vi "fetch frame gige DB1605.vi"() -> ()   [LabVIEW 2015]
uses:
  <vilib>/Utility/miscctls.llb/LV3DPointTypeDef.ctl
  <vilib>/Utility/miscctls.llb/LVRGBAColorTypeDef.ctl
  <vilib>/Utility/importsl/GetValueByPointer/datatype.ctl
  <vilib>/Utility/importsl/GetValueByPointer/GetValueByPointer.xnode
  <userlib>/Mv3dRgbd/Mv3dRgbd.lvlib
  <vilib>/picture/3D Picture Control/NI_3D Picture Control.lvlib
  <userlib>/Mv3dRgbdEx/Mv3dRgbdEx.lvlib
panel:
  in  "InputType":cluster{string}
  out "Output":cluster{string}
  out "pstCalibInfo out":T1
  out "handle out":u32
  out "function return":i32
  in  "nCoordinateType":u32
  out "pDeviceCount out 4":u32
  out "pstGigeDeviceInfo out 3":T2
  out "start handle out":u32
  in  "?":enum32{"RGBD", "点云"}(tab)
  out "二维图片":picture
  out "Depth":i16[][](graph)
  out "init function":i32
  out "get list return 3":i32
  out "open gige function 2":i32
  out "start function 2":i32
  out "fetchframe function":i32
  out "stop function":i32
  out "depthtocloud return":i32
  out "close function":i32
  out "release function":i32
  in  "?":bool
  out "MV3D_RGBD_GigEDEVICE_INFO out 3":T3(array[cluster])
  in  "设备索引":i32=5
  out "?":refnum<vi>(3d-picture)
  in  "Name":string="XYZ轴" caption="名称"
  out "大小":i32
  out "x+1":i32
  out "close handle out":u32
  out "stop handle out":u32
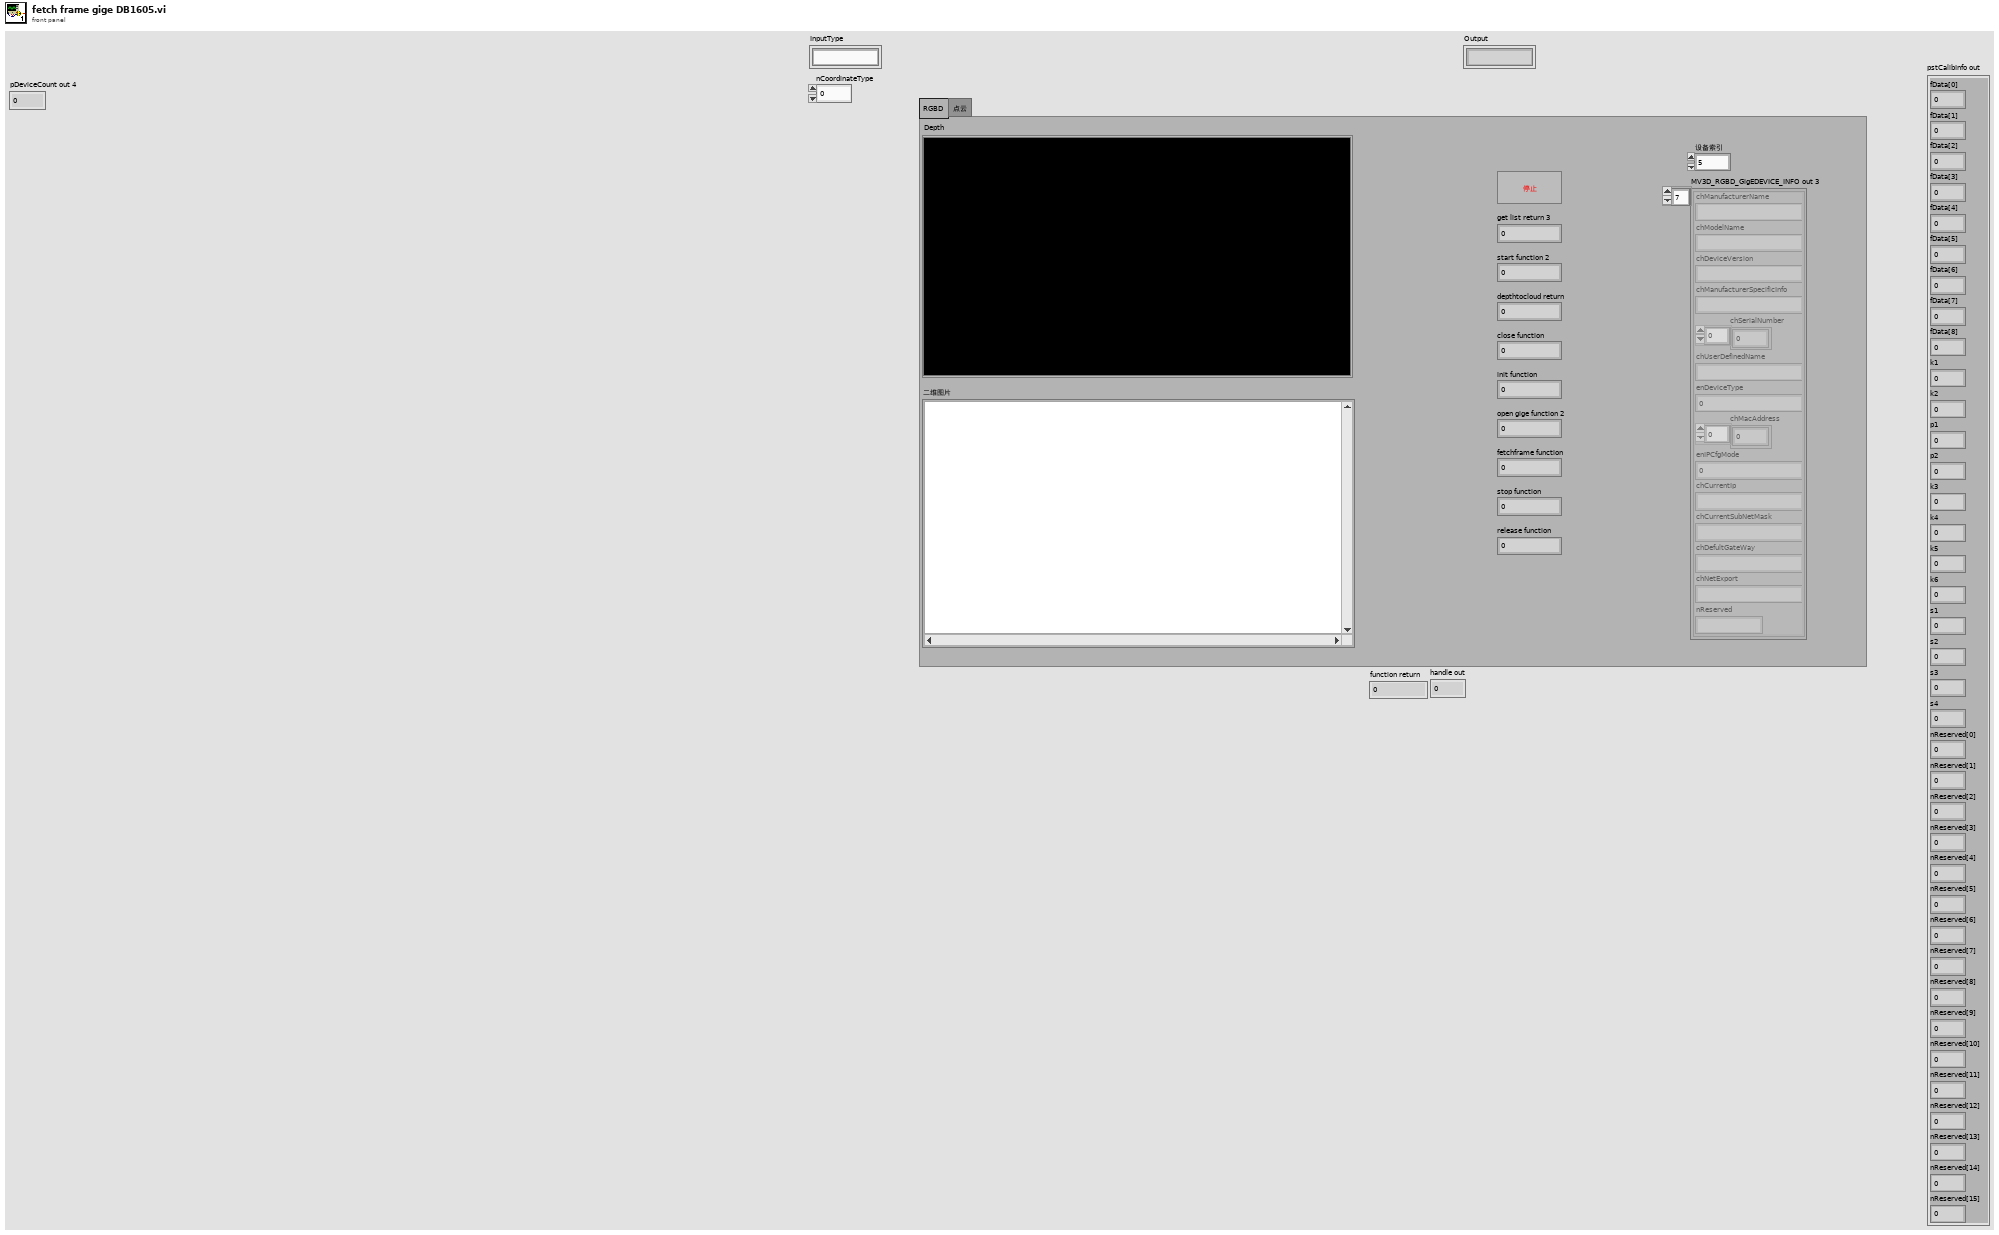
[diagram p1: front panel]
types:
  T1 = cluster{"fData[0]":sgl, "fData[1]":sgl, "fData[2]":sgl, "fData[3]":sgl, "fData[4]":sgl, "fData[5]":sgl, "fData[6]":sgl, "fData[7]":sgl, "fData[8]":sgl, "k1":sgl, "k2":sgl, "p1":sgl, "p2":sgl, "k3":sgl, "k4":sgl, "k5":sgl, "k6":sgl, "s1":sgl, "s2":sgl, "s3":sgl, "s4":sgl, "nReserved[0]":u8, "nReserved[1]":u8, "nReserved[2]":u8, "nReserved[3]":u8, "nReserved[4]":u8, "nReserved[5]":u8, "nReserved[6]":u8, "nReserved[7]":u8, "nReserved[8]":u8, "nReserved[9]":u8, "nReserved[10]":u8, "nReserved[11]":u8, "nReserved[12]":u8, "nReserved[13]":u8, "nReserved[14]":u8, "nReserved[15]":u8}
  T2 = cluster{"chManufacturerName[0]":i8, "chManufacturerName[1]":i8, "chManufacturerName[2]":i8, "chManufacturerName[3]":i8, "chManufacturerName[4]":i8, "chManufacturerName[5]":i8, "chManufacturerName[6]":i8, "chManufacturerName[7]":i8, "chManufacturerName[8]":i8, "chManufacturerName[9]":i8, "chManufacturerName[10]":i8, "chManufacturerName[11]":i8, "chManufacturerName[12]":i8, "chManufacturerName[13]":i8, "chManufacturerName[14]":i8, "chManufacturerName[15]":i8, "chManufacturerName[16]":i8, "chManufacturerName[17]":i8, "chManufacturerName[18]":i8, "chManufacturerName[19]":i8, "chManufacturerName[20]":i8, "chManufacturerName[21]":i8, "chManufacturerName[22]":i8, "chManufacturerName[23]":i8, "chManufacturerName[24]":i8, "chManufacturerName[25]":i8, "chManufacturerName[26]":i8, "chManufacturerName[27]":i8, "chManufacturerName[28]":i8, "chManufacturerName[29]":i8, "chManufacturerName[30]":i8, "chManufacturerName[31]":i8, "chModelName[0]":i8, "chModelName[1]":i8, "chModelName[2]":i8, "chModelName[3]":i8, "chModelName[4]":i8, "chModelName[5]":i8, "chModelName[6]":i8, "chModelName[7]":i8, "chModelName[8]":i8, "chModelName[9]":i8, "chModelName[10]":i8, "chModelName[11]":i8, "chModelName[12]":i8, "chModelName[13]":i8, "chModelName[14]":i8, "chModelName[15]":i8, "chModelName[16]":i8, "chModelName[17]":i8, "chModelName[18]":i8, "chModelName[19]":i8, "chModelName[20]":i8, "chModelName[21]":i8, "chModelName[22]":i8, "chModelName[23]":i8, "chModelName[24]":i8, "chModelName[25]":i8, "chModelName[26]":i8, "chModelName[27]":i8, "chModelName[28]":i8, "chModelName[29]":i8, "chModelName[30]":i8, "chModelName[31]":i8, "chDeviceVersion[0]":i8, "chDeviceVersion[1]":i8, "chDeviceVersion[2]":i8, "chDeviceVersion[3]":i8, "chDeviceVersion[4]":i8, "chDeviceVersion[5]":i8, "chDeviceVersion[6]":i8, "chDeviceVersion[7]":i8, "chDeviceVersion[8]":i8, "chDeviceVersion[9]":i8, "chDeviceVersion[10]":i8, "chDeviceVersion[11]":i8, "chDeviceVersion[12]":i8, "chDeviceVersion[13]":i8, "chDeviceVersion[14]":i8, "chDeviceVersion[15]":i8, "chDeviceVersion[16]":i8, "chDeviceVersion[17]":i8, "chDeviceVersion[18]":i8, "chDeviceVersion[19]":i8, "chDeviceVersion[20]":i8, "chDeviceVersion[21]":i8, "chDeviceVersion[22]":i8, "chDeviceVersion[23]":i8, "chDeviceVersion[24]":i8, "chDeviceVersion[25]":i8, "chDeviceVersion[26]":i8, "chDeviceVersion[27]":i8, "chDeviceVersion[28]":i8, "chDeviceVersion[29]":i8, "chDeviceVersion[30]":i8, "chDeviceVersion[31]":i8, "chManufacturerSpecificInfo[0]":i8, "chManufacturerSpecificInfo[1]":i8, "chManufacturerSpecificInfo[2]":i8, "chManufacturerSpecificInfo[3]":i8, "chManufacturerSpecificInfo[4]":i8, "chManufacturerSpecificInfo[5]":i8, "chManufacturerSpecificInfo[6]":i8, "chManufacturerSpecificInfo[7]":i8, "chManufacturerSpecificInfo[8]":i8, "chManufacturerSpecificInfo[9]":i8, "chManufacturerSpecificInfo[10]":i8, "chManufacturerSpecificInfo[11]":i8, "chManufacturerSpecificInfo[12]":i8, "chManufacturerSpecificInfo[13]":i8, "chManufacturerSpecificInfo[14]":i8, "chManufacturerSpecificInfo[15]":i8, "chManufacturerSpecificInfo[16]":i8, "chManufacturerSpecificInfo[17]":i8, "chManufacturerSpecificInfo[18]":i8, "chManufacturerSpecificInfo[19]":i8, "chManufacturerSpecificInfo[20]":i8, "chManufacturerSpecificInfo[21]":i8, "chManufacturerSpecificInfo[22]":i8, "chManufacturerSpecificInfo[23]":i8, "chManufacturerSpecificInfo[24]":i8, "chManufacturerSpecificInfo[25]":i8, "chManufacturerSpecificInfo[26]":i8, "chManufacturerSpecificInfo[27]":i8, "chManufacturerSpecificInfo[28]":i8, "chManufacturerSpecificInfo[29]":i8, "chManufacturerSpecificInfo[30]":i8, "chManufacturerSpecificInfo[31]":i8, "chManufacturerSpecificInfo[32]":i8, "chManufacturerSpecificInfo[33]":i8, "chManufacturerSpecificInfo[34]":i8, "chManufacturerSpecificInfo[35]":i8, "chManufacturerSpecificInfo[36]":i8, "chManufacturerSpecificInfo[37]":i8, "chManufacturerSpecificInfo[38]":i8, "chManufacturerSpecificInfo[39]":i8, "chManufacturerSpecificInfo[40]":i8, "chManufacturerSpecificInfo[41]":i8, "chManufacturerSpecificInfo[42]":i8, "chManufacturerSpecificInfo[43]":i8, "chManufacturerSpecificInfo[44]":i8, "chManufacturerSpecificInfo[45]":i8, "chManufacturerSpecificInfo[46]":i8, "chManufacturerSpecificInfo[47]":i8, "chSerialNumber[0]":i8, "chSerialNumber[1]":i8, "chSerialNumber[2]":i8, "chSerialNumber[3]":i8, "chSerialNumber[4]":i8, "chSerialNumber[5]":i8, "chSerialNumber[6]":i8, "chSerialNumber[7]":i8, "chSerialNumber[8]":i8, "chSerialNumber[9]":i8, "chSerialNumber[10]":i8, "chSerialNumber[11]":i8, "chSerialNumber[12]":i8, "chSerialNumber[13]":i8, "chSerialNumber[14]":i8, "chSerialNumber[15]":i8, "chUserDefinedName[0]":i8, "chUserDefinedName[1]":i8, "chUserDefinedName[2]":i8, "chUserDefinedName[3]":i8, "chUserDefinedName[4]":i8, "chUserDefinedName[5]":i8, "chUserDefinedName[6]":i8, "chUserDefinedName[7]":i8, "chUserDefinedName[8]":i8, "chUserDefinedName[9]":i8, "chUserDefinedName[10]":i8, "chUserDefinedName[11]":i8, "chUserDefinedName[12]":i8, "chUserDefinedName[13]":i8, "chUserDefinedName[14]":i8, "chUserDefinedName[15]":i8, "enDeviceType":i32, "chMacAddress[0]":u8, "chMacAddress[1]":u8, "chMacAddress[2]":u8, "chMacAddress[3]":u8, "chMacAddress[4]":u8, "chMacAddress[5]":u8, "chMacAddress[6]":u8, "chMacAddress[7]":u8, "enIPCfgMode":i32, "chCurrentIp[0]":i8, "chCurrentIp[1]":i8, "chCurrentIp[2]":i8, "chCurrentIp[3]":i8, "chCurrentIp[4]":i8, "chCurrentIp[5]":i8, "chCurrentIp[6]":i8, "chCurrentIp[7]":i8, "chCurrentIp[8]":i8, "chCurrentIp[9]":i8, "chCurrentIp[10]":i8, "chCurrentIp[11]":i8, "chCurrentIp[12]":i8, "chCurrentIp[13]":i8, "chCurrentIp[14]":i8, "chCurrentIp[15]":i8, "chCurrentSubNetMask[0]":i8, "chCurrentSubNetMask[1]":i8, "chCurrentSubNetMask[2]":i8, "chCurrentSubNetMask[3]":i8, "chCurrentSubNetMask[4]":i8, "chCurrentSubNetMask[5]":i8, "chCurrentSubNetMask[6]":i8, "chCurrentSubNetMask[7]":i8, "chCurrentSubNetMask[8]":i8, "chCurrentSubNetMask[9]":i8, "chCurrentSubNetMask[10]":i8, "chCurrentSubNetMask[11]":i8, "chCurrentSubNetMask[12]":i8, "chCurrentSubNetMask[13]":i8, "chCurrentSubNetMask[14]":i8, "chCurrentSubNetMask[15]":i8, "chDefultGateWay[0]":i8, "chDefultGateWay[1]":i8, "chDefultGateWay[2]":i8, "chDefultGateWay[3]":i8, "chDefultGateWay[4]":i8, "chDefultGateWay[5]":i8, "chDefultGateWay[6]":i8, "chDefultGateWay[7]":i8, "chDefultGateWay[8]":i8, "chDefultGateWay[9]":i8, "chDefultGateWay[10]":i8, "chDefultGateWay[11]":i8, "chDefultGateWay[12]":i8, "chDefultGateWay[13]":i8, "chDefultGateWay[14]":i8, "chDefultGateWay[15]":i8, "chNetExport[0]":i8, "chNetExport[1]":i8, "chNetExport[2]":i8, "chNetExport[3]":i8, "chNetExport[4]":i8, "chNetExport[5]":i8, "chNetExport[6]":i8, "chNetExport[7]":i8, "chNetExport[8]":i8, "chNetExport[9]":i8, "chNetExport[10]":i8, "chNetExport[11]":i8, "chNetExport[12]":i8, "chNetExport[13]":i8, "chNetExport[14]":i8, "chNetExport[15]":i8, "nReserved[0]":u8, "nReserved[1]":u8, "nReserved[2]":u8, "nReserved[3]":u8, "nReserved[4]":u8, "nReserved[5]":u8, "nReserved[6]":u8, "nReserved[7]":u8, "nReserved[8]":u8, "nReserved[9]":u8, "nReserved[10]":u8, "nReserved[11]":u8, "nReserved[12]":u8, "nReserved[13]":u8, "nReserved[14]":u8, "nReserved[15]":u8}
  T3 = cluster{"chManufacturerName":string, "chModelName":string, "chDeviceVersion":string, "chManufacturerSpecificInfo":string, "chSerialNumber":u8[], "chUserDefinedName":string, "enDeviceType":i32, "chMacAddress":u8[], "enIPCfgMode":i32, "chCurrentIp":string, "chCurrentSubNetMask":string, "chDefultGateWay":string, "chNetExport":string, "nReserved":string}[]
  T4 = typedef "LV3DPointTypeDef.ctl" = cluster{"X":sgl, "Y":sgl, "Z":sgl}
  T5 = typedef "LVRGBAColorTypeDef.ctl" = cluster{"Red":sgl, "Green":sgl, "Blue":sgl, "Alpha":sgl}
  T6 = cluster{"Red":sgl, "Green":sgl, "Blue":sgl, "Alpha":sgl}
  T7 = enum32{"pack1", "pack2", "pack4", "pack8", "pack16"}
  T8 = enum16{"Overall", "Per Primitive", "Per Vertex", "Binding Off"}
  T9 = enum16{"Points", "Lines", "Line Strip", "Line Loop", "Triangles", "Triangle Strip", "Triangle Fan", "Quads", "Quad Strip", "Polygon"}
  T10 = cluster{"chManufacturerName[0]":i8, "chManufacturerName[1]":i8, "chManufacturerName[2]":i8, "chManufacturerName[3]":i8, "chManufacturerName[4]":i8, "chManufacturerName[5]":i8, "chManufacturerName[6]":i8, "chManufacturerName[7]":i8, "chManufacturerName[8]":i8, "chManufacturerName[9]":i8, "chManufacturerName[10]":i8, "chManufacturerName[11]":i8, "chManufacturerName[12]":i8, "chManufacturerName[13]":i8, "chManufacturerName[14]":i8, "chManufacturerName[15]":i8, "chManufacturerName[16]":i8, "chManufacturerName[17]":i8, "chManufacturerName[18]":i8, "chManufacturerName[19]":i8, "chManufacturerName[20]":i8, "chManufacturerName[21]":i8, "chManufacturerName[22]":i8, "chManufacturerName[23]":i8, "chManufacturerName[24]":i8, "chManufacturerName[25]":i8, "chManufacturerName[26]":i8, "chManufacturerName[27]":i8, "chManufacturerName[28]":i8, "chManufacturerName[29]":i8, "chManufacturerName[30]":i8, "chManufacturerName[31]":i8, "chModelName[0]":i8, "chModelName[1]":i8, "chModelName[2]":i8, "chModelName[3]":i8, "chModelName[4]":i8, "chModelName[5]":i8, "chModelName[6]":i8, "chModelName[7]":i8, "chModelName[8]":i8, "chModelName[9]":i8, "chModelName[10]":i8, "chModelName[11]":i8, "chModelName[12]":i8, "chModelName[13]":i8, "chModelName[14]":i8, "chModelName[15]":i8, "chModelName[16]":i8, "chModelName[17]":i8, "chModelName[18]":i8, "chModelName[19]":i8, "chModelName[20]":i8, "chModelName[21]":i8, "chModelName[22]":i8, "chModelName[23]":i8, "chModelName[24]":i8, "chModelName[25]":i8, "chModelName[26]":i8, "chModelName[27]":i8, "chModelName[28]":i8, "chModelName[29]":i8, "chModelName[30]":i8, "chModelName[31]":i8, "chDeviceVersion[0]":i8, "chDeviceVersion[1]":i8, "chDeviceVersion[2]":i8, "chDeviceVersion[3]":i8, "chDeviceVersion[4]":i8, "chDeviceVersion[5]":i8, "chDeviceVersion[6]":i8, "chDeviceVersion[7]":i8, "chDeviceVersion[8]":i8, "chDeviceVersion[9]":i8, "chDeviceVersion[10]":i8, "chDeviceVersion[11]":i8, "chDeviceVersion[12]":i8, "chDeviceVersion[13]":i8, "chDeviceVersion[14]":i8, "chDeviceVersion[15]":i8, "chDeviceVersion[16]":i8, "chDeviceVersion[17]":i8, "chDeviceVersion[18]":i8, "chDeviceVersion[19]":i8, "chDeviceVersion[20]":i8, "chDeviceVersion[21]":i8, "chDeviceVersion[22]":i8, "chDeviceVersion[23]":i8, "chDeviceVersion[24]":i8, "chDeviceVersion[25]":i8, "chDeviceVersion[26]":i8, "chDeviceVersion[27]":i8, "chDeviceVersion[28]":i8, "chDeviceVersion[29]":i8, "chDeviceVersion[30]":i8, "chDeviceVersion[31]":i8, "chManufacturerSpecificInfo[0]":i8, "chManufacturerSpecificInfo[1]":i8, "chManufacturerSpecificInfo[2]":i8, "chManufacturerSpecificInfo[3]":i8, "chManufacturerSpecificInfo[4]":i8, "chManufacturerSpecificInfo[5]":i8, "chManufacturerSpecificInfo[6]":i8, "chManufacturerSpecificInfo[7]":i8, "chManufacturerSpecificInfo[8]":i8, "chManufacturerSpecificInfo[9]":i8, "chManufacturerSpecificInfo[10]":i8, "chManufacturerSpecificInfo[11]":i8, "chManufacturerSpecificInfo[12]":i8, "chManufacturerSpecificInfo[13]":i8, "chManufacturerSpecificInfo[14]":i8, "chManufacturerSpecificInfo[15]":i8, "chManufacturerSpecificInfo[16]":i8, "chManufacturerSpecificInfo[17]":i8, "chManufacturerSpecificInfo[18]":i8, "chManufacturerSpecificInfo[19]":i8, "chManufacturerSpecificInfo[20]":i8, "chManufacturerSpecificInfo[21]":i8, "chManufacturerSpecificInfo[22]":i8, "chManufacturerSpecificInfo[23]":i8, "chManufacturerSpecificInfo[24]":i8, "chManufacturerSpecificInfo[25]":i8, "chManufacturerSpecificInfo[26]":i8, "chManufacturerSpecificInfo[27]":i8, "chManufacturerSpecificInfo[28]":i8, "chManufacturerSpecificInfo[29]":i8, "chManufacturerSpecificInfo[30]":i8, "chManufacturerSpecificInfo[31]":i8, "chManufacturerSpecificInfo[32]":i8, "chManufacturerSpecificInfo[33]":i8, "chManufacturerSpecificInfo[34]":i8, "chManufacturerSpecificInfo[35]":i8, "chManufacturerSpecificInfo[36]":i8, "chManufacturerSpecificInfo[37]":i8, "chManufacturerSpecificInfo[38]":i8, "chManufacturerSpecificInfo[39]":i8, "chManufacturerSpecificInfo[40]":i8, "chManufacturerSpecificInfo[41]":i8, "chManufacturerSpecificInfo[42]":i8, "chManufacturerSpecificInfo[43]":i8, "chManufacturerSpecificInfo[44]":i8, "chManufacturerSpecificInfo[45]":i8, "chManufacturerSpecificInfo[46]":i8, "chManufacturerSpecificInfo[47]":i8, "chSerialNumber[0]":i8, "chSerialNumber[1]":i8, "chSerialNumber[2]":i8, "chSerialNumber[3]":i8, "chSerialNumber[4]":i8, "chSerialNumber[5]":i8, "chSerialNumber[6]":i8, "chSerialNumber[7]":i8, "chSerialNumber[8]":i8, "chSerialNumber[9]":i8, "chSerialNumber[10]":i8, "chSerialNumber[11]":i8, "chSerialNumber[12]":i8, "chSerialNumber[13]":i8, "chSerialNumber[14]":i8, "chSerialNumber[15]":i8, "chUserDefinedName[0]":i8, "chUserDefinedName[1]":i8, "chUserDefinedName[2]":i8, "chUserDefinedName[3]":i8, "chUserDefinedName[4]":i8, "chUserDefinedName[5]":i8, "chUserDefinedName[6]":i8, "chUserDefinedName[7]":i8, "chUserDefinedName[8]":i8, "chUserDefinedName[9]":i8, "chUserDefinedName[10]":i8, "chUserDefinedName[11]":i8, "chUserDefinedName[12]":i8, "chUserDefinedName[13]":i8, "chUserDefinedName[14]":i8, "chUserDefinedName[15]":i8, "enDeviceType":i32, "chMacAddress[0]":u8, "chMacAddress[1]":u8, "chMacAddress[2]":u8, "chMacAddress[3]":u8, "chMacAddress[4]":u8, "chMacAddress[5]":u8, "chMacAddress[6]":u8, "chMacAddress[7]":u8, "enIPCfgMode":i32, "chCurrentIp[0]":i8, "chCurrentIp[1]":i8, "chCurrentIp[2]":i8, "chCurrentIp[3]":i8, "chCurrentIp[4]":i8, "chCurrentIp[5]":i8, "chCurrentIp[6]":i8, "chCurrentIp[7]":i8, "chCurrentIp[8]":i8, "chCurrentIp[9]":i8, "chCurrentIp[10]":i8, "chCurrentIp[11]":i8, "chCurrentIp[12]":i8, "chCurrentIp[13]":i8, "chCurrentIp[14]":i8, "chCurrentIp[15]":i8, "chCurrentSubNetMask[0]":i8, "chCurrentSubNetMask[1]":i8, "chCurrentSubNetMask[2]":i8, "chCurrentSubNetMask[3]":i8, "chCurrentSubNetMask[4]":i8, "chCurrentSubNetMask[5]":i8, "chCurrentSubNetMask[6]":i8, "chCurrentSubNetMask[7]":i8, "chCurrentSubNetMask[8]":i8, "chCurrentSubNetMask[9]":i8, "chCurrentSubNetMask[10]":i8, "chCurrentSubNetMask[11]":i8, "chCurrentSubNetMask[12]":i8, "chCurrentSubNetMask[13]":i8, "chCurrentSubNetMask[14]":i8, "chCurrentSubNetMask[15]":i8, "chDefultGateWay[0]":i8, "chDefultGateWay[1]":i8, "chDefultGateWay[2]":i8, "chDefultGateWay[3]":i8, "chDefultGateWay[4]":i8, "chDefultGateWay[5]":i8, "chDefultGateWay[6]":i8, "chDefultGateWay[7]":i8, "chDefultGateWay[8]":i8, "chDefultGateWay[9]":i8, "chDefultGateWay[10]":i8, "chDefultGateWay[11]":i8, "chDefultGateWay[12]":i8, "chDefultGateWay[13]":i8, "chDefultGateWay[14]":i8, "chDefultGateWay[15]":i8, "chNetExport[0]":i8, "chNetExport[1]":i8, "chNetExport[2]":i8, "chNetExport[3]":i8, "chNetExport[4]":i8, "chNetExport[5]":i8, "chNetExport[6]":i8, "chNetExport[7]":i8, "chNetExport[8]":i8, "chNetExport[9]":i8, "chNetExport[10]":i8, "chNetExport[11]":i8, "chNetExport[12]":i8, "chNetExport[13]":i8, "chNetExport[14]":i8, "chNetExport[15]":i8, "nReserved[0]":u8, "nReserved[1]":u8, "nReserved[2]":u8, "nReserved[3]":u8, "nReserved[4]":u8, "nReserved[5]":u8, "nReserved[6]":u8, "nReserved[7]":u8, "nReserved[8]":u8, "nReserved[9]":u8, "nReserved[10]":u8, "nReserved[11]":u8, "nReserved[12]":u8, "nReserved[13]":u8, "nReserved[14]":u8, "nReserved[15]":u8}[]
  T11 = cluster{"nImageCount":u64, "MV3D_RGBD_IMAGE_DATA[0]":cluster{"enImageType":i32, "nWidth":u32, "nHeight":u32, "pData":u32, "nDataLen":u32, "nFrameNum":u32, "nTimeStamp":i64, "nReserved[0]":u8, "nReserved[1]":u8, "nReserved[2]":u8, "nReserved[3]":u8, "nReserved[4]":u8, "nReserved[5]":u8, "nReserved[6]":u8, "nReserved[7]":u8, "nReserved[8]":u8, "nReserved[9]":u8, "nReserved[10]":u8, "nReserved[11]":u8, "nReserved[12]":u8, "nReserved[13]":u8, "nReserved[14]":u8, "nReserved[15]":u8}, "MV3D_RGBD_IMAGE_DATA[1]":cluster{"enImageType":i32, "nWidth":u32, "nHeight":u32, "pData":u32, "nDataLen":u32, "nFrameNum":u32, "nTimeStamp":i64, "nReserved[0]":u8, "nReserved[1]":u8, "nReserved[2]":u8, "nReserved[3]":u8, "nReserved[4]":u8, "nReserved[5]":u8, "nReserved[6]":u8, "nReserved[7]":u8, "nReserved[8]":u8, "nReserved[9]":u8, "nReserved[10]":u8, "nReserved[11]":u8, "nReserved[12]":u8, "nReserved[13]":u8, "nReserved[14]":u8, "nReserved[15]":u8}, "MV3D_RGBD_IMAGE_DATA[2]":cluster{"enImageType":i32, "nWidth":u32, "nHeight":u32, "pData":u32, "nDataLen":u32, "nFrameNum":u32, "nTimeStamp":i64, "nReserved[0]":u8, "nReserved[1]":u8, "nReserved[2]":u8, "nReserved[3]":u8, "nReserved[4]":u8, "nReserved[5]":u8, "nReserved[6]":u8, "nReserved[7]":u8, "nReserved[8]":u8, "nReserved[9]":u8, "nReserved[10]":u8, "nReserved[11]":u8, "nReserved[12]":u8, "nReserved[13]":u8, "nReserved[14]":u8, "nReserved[15]":u8}, "MV3D_RGBD_IMAGE_DATA[3]":cluster{"enImageType":i32, "nWidth":u32, "nHeight":u32, "pData":u32, "nDataLen":u32, "nFrameNum":u32, "nTimeStamp":i64, "nReserved[0]":u8, "nReserved[1]":u8, "nReserved[2]":u8, "nReserved[3]":u8, "nReserved[4]":u8, "nReserved[5]":u8, "nReserved[6]":u8, "nReserved[7]":u8, "nReserved[8]":u8, "nReserved[9]":u8, "nReserved[10]":u8, "nReserved[11]":u8, "nReserved[12]":u8, "nReserved[13]":u8, "nReserved[14]":u8, "nReserved[15]":u8}, "MV3D_RGBD_IMAGE_DATA[4]":cluster{"enImageType":i32, "nWidth":u32, "nHeight":u32, "pData":u32, "nDataLen":u32, "nFrameNum":u32, "nTimeStamp":i64, "nReserved[0]":u8, "nReserved[1]":u8, "nReserved[2]":u8, "nReserved[3]":u8, "nReserved[4]":u8, "nReserved[5]":u8, "nReserved[6]":u8, "nReserved[7]":u8, "nReserved[8]":u8, "nReserved[9]":u8, "nReserved[10]":u8, "nReserved[11]":u8, "nReserved[12]":u8, "nReserved[13]":u8, "nReserved[14]":u8, "nReserved[15]":u8}, "MV3D_RGBD_IMAGE_DATA[5]":cluster{"enImageType":i32, "nWidth":u32, "nHeight":u32, "pData":u32, "nDataLen":u32, "nFrameNum":u32, "nTimeStamp":i64, "nReserved[0]":u8, "nReserved[1]":u8, "nReserved[2]":u8, "nReserved[3]":u8, "nReserved[4]":u8, "nReserved[5]":u8, "nReserved[6]":u8, "nReserved[7]":u8, "nReserved[8]":u8, "nReserved[9]":u8, "nReserved[10]":u8, "nReserved[11]":u8, "nReserved[12]":u8, "nReserved[13]":u8, "nReserved[14]":u8, "nReserved[15]":u8}, "MV3D_RGBD_IMAGE_DATA[6]":cluster{"enImageType":i32, "nWidth":u32, "nHeight":u32, "pData":u32, "nDataLen":u32, "nFrameNum":u32, "nTimeStamp":i64, "nReserved[0]":u8, "nReserved[1]":u8, "nReserved[2]":u8, "nReserved[3]":u8, "nReserved[4]":u8, "nReserved[5]":u8, "nReserved[6]":u8, "nReserved[7]":u8, "nReserved[8]":u8, "nReserved[9]":u8, "nReserved[10]":u8, "nReserved[11]":u8, "nReserved[12]":u8, "nReserved[13]":u8, "nReserved[14]":u8, "nReserved[15]":u8}, "MV3D_RGBD_IMAGE_DATA[7]":cluster{"enImageType":i32, "nWidth":u32, "nHeight":u32, "pData":u32, "nDataLen":u32, "nFrameNum":u32, "nTimeStamp":i64, "nReserved[0]":u8, "nReserved[1]":u8, "nReserved[2]":u8, "nReserved[3]":u8, "nReserved[4]":u8, "nReserved[5]":u8, "nReserved[6]":u8, "nReserved[7]":u8, "nReserved[8]":u8, "nReserved[9]":u8, "nReserved[10]":u8, "nReserved[11]":u8, "nReserved[12]":u8, "nReserved[13]":u8, "nReserved[14]":u8, "nReserved[15]":u8}, "MV3D_RGBD_IMAGE_DATA[8]":cluster{"enImageType":i32, "nWidth":u32, "nHeight":u32, "pData":u32, "nDataLen":u32, "nFrameNum":u32, "nTimeStamp":i64, "nReserved[0]":u8, "nReserved[1]":u8, "nReserved[2]":u8, "nReserved[3]":u8, "nReserved[4]":u8, "nReserved[5]":u8, "nReserved[6]":u8, "nReserved[7]":u8, "nReserved[8]":u8, "nReserved[9]":u8, "nReserved[10]":u8, "nReserved[11]":u8, "nReserved[12]":u8, "nReserved[13]":u8, "nReserved[14]":u8, "nReserved[15]":u8}, "MV3D_RGBD_IMAGE_DATA[9]":cluster{"enImageType":i32, "nWidth":u32, "nHeight":u32, "pData":u32, "nDataLen":u32, "nFrameNum":u32, "nTimeStamp":i64, "nReserved[0]":u8, "nReserved[1]":u8, "nReserved[2]":u8, "nReserved[3]":u8, "nReserved[4]":u8, "nReserved[5]":u8, "nReserved[6]":u8, "nReserved[7]":u8, "nReserved[8]":u8, "nReserved[9]":u8, "nReserved[10]":u8, "nReserved[11]":u8, "nReserved[12]":u8, "nReserved[13]":u8, "nReserved[14]":u8, "nReserved[15]":u8}, "nReserved[0]":u8, "nReserved[1]":u8, "nReserved[2]":u8, "nReserved[3]":u8, "nReserved[4]":u8, "nReserved[5]":u8, "nReserved[6]":u8, "nReserved[7]":u8, "nReserved[8]":u8, "nReserved[9]":u8, "nReserved[10]":u8, "nReserved[11]":u8, "nReserved[12]":u8, "nReserved[13]":u8, "nReserved[14]":u8, "nReserved[15]":u8}
  T12 = cluster{"enImageType":i32, "nWidth":u32, "nHeight":u32, "pData":u32, "nDataLen":u32, "nFrameNum":u32, "nTimeStamp":i64, "nReserved[0]":u8, "nReserved[1]":u8, "nReserved[2]":u8, "nReserved[3]":u8, "nReserved[4]":u8, "nReserved[5]":u8, "nReserved[6]":u8, "nReserved[7]":u8, "nReserved[8]":u8, "nReserved[9]":u8, "nReserved[10]":u8, "nReserved[11]":u8, "nReserved[12]":u8, "nReserved[13]":u8, "nReserved[14]":u8, "nReserved[15]":u8}
  T13 = typedef "imagedata.ctl" = cluster{"image type":i32, "image depth":i32, "image":u8[], "mask":u8[], "colors":u32[], "Rectangle":cluster{"left":i16, "top":i16, "right":i16, "bottom":i16}}
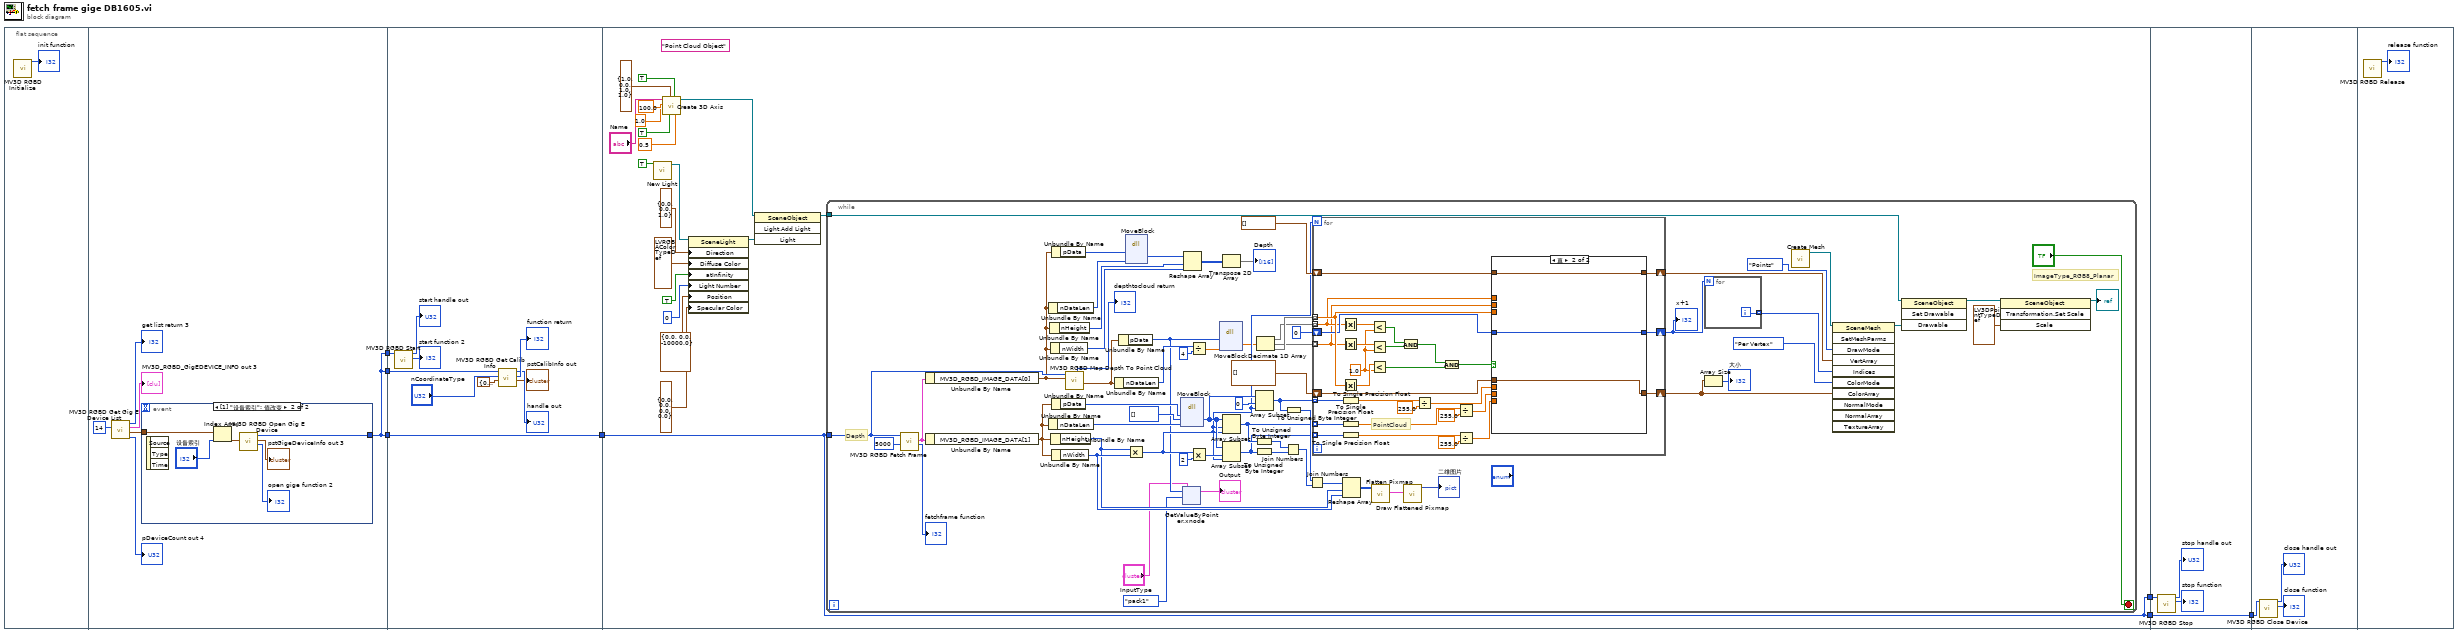
[diagram p0: block diagram]
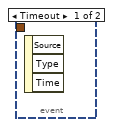
[diagram p2: hidden frame]
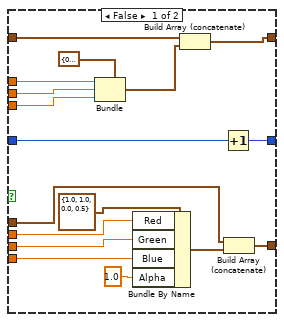
[diagram p3: hidden frame]
diagram:
  n1 = flat-sequence {
    tunnel: [w9] -> w4
    tunnel: [w9] -> w3
    tunnel: [w9] -> w1
    tunnel: w4 -> [w28]
    tunnel: w3 -> [w27]
    tunnel: [w27] -> w2
    tunnel: w1 -> [w26]
    tunnel: [w49] -> w6
    tunnel: [w49] -> w5
    tunnel: w2 -> [w49]
    tunnel: [w179] -> w7
    tunnel: w6 -> [w179]
    tunnel: w5 -> [w180]
    tunnel: w7 -> [w183]
    frame #0 {
      n2 = call <userlib>:"MV3D RGBD Initialize.vi"() -> ("function return"=→"init function":i32)  [unwired: 11 in]
    }
    frame #1 {
      n3 = call <userlib>:"MV3D RGBD Get Gig E Device List.vi"("nMaxDeviceCount"=u32 14) -> ("pDeviceCount out"=→"pDeviceCount out 4":u32, "MV3D_RGBD_GigEDEVICE_ByteINFO out"=w10:T10, "MV3D_RGBD_GigEDEVICE_INFO out"=→"MV3D_RGBD_GigEDEVICE_INFO out 3":T3, "function return"=→"get list return 3":i32)  [unwired: 7 in]
      n4 = event shown="[1] \"设备索引\": 值改变" {
        selector: _ -> [_ _]
        dyn-events: _ -> [_ _]
        timeout: _ -> [_ _]
        tunnel: w10 -> [_ w16]
        tunnel: [_ w15] -> w9
        event Timeout {
          n5 = event-data() -> ()  [unwired: 1 in, 3 out]
        }
        event "设备索引": Value Change {
          n6 = event-data() -> ()  [unwired: 1 in, 3 out]
          n7 = Index Array(array=w16, index="设备索引") -> (element=w18:T2)
          n8 = call <userlib>:"MV3D RGBD Open Gig E Device.vi"("pstGigeDeviceInfo 2"=w18) -> ("handle out"=w15:u32, "pstGigeDeviceInfo out"=→"pstGigeDeviceInfo out 3":T2, "function return"=→"open gige function 2":i32)  [unwired: 7 in]
        }
      }
    }
    frame #2 {
      n9 = call <userlib>:"MV3D RGBD Start.vi"("handle"=w28) -> ("function return"=→"start function 2":i32, "handle out"=→"start handle out":u32)  [unwired: 9 in]
      n10 = call <userlib>:"MV3D RGBD Get Calib Info.vi"("pstCalibInfo"=T1 {"fData[0]"=0.0, "fData[1]"=0.0, "fData[2]"=0.0, "fData[3]"=0.0, "fData[4]"=0.0, "fData[5]"=0.0, "fData[6]"=0.0, "fData[7]"=0.0, "fData[8]"=0.0, "k1"=0.0, "k2"=0.0, "p1"=0.0, "p2"=0.0, "k3"=0.0, "k4"=0.0, "k5"=0.0, "k6"=0.0, "s1"=0.0, "s2"=0.0, "s3"=0.0, "s4"=0.0, "nReserved[0]"=0, "nReserved[1]"=0, "nReserved[2]"=0, "nReserved[3]"=0, "nReserved[4]"=0, "nReserved[5]"=0, "nReserved[6]"=0, "nReserved[7]"=0, "nReserved[8]"=0, "nReserved[9]"=0, "nReserved[10]"=0, "nReserved[11]"=0, "nReserved[12]"=0, "nReserved[13]"=0, "nReserved[14]"=0, "nReserved[15]"=0}, "nCoordinateType"="nCoordinateType", "handle"=w26) -> ("pstCalibInfo out"=→"pstCalibInfo out":T1, "function return"=→"function return":i32, "handle out"=→"handle out":u32)  [unwired: 6 in]
    }
    frame #3 {
      (unwired) "Point Cloud Object" ("Name")
      n11 = call <vilib>:"New Light.vi"("At Infinity"=TRUE) -> ("New Light Refnum"=w37:refnum<vi>)  [unwired: 9 in, 1 out]
      n12 = call <vilib>:"Create 3D Axis.vi"("Character Size"=sgl 0.5, "Half plane?"=TRUE, "Axis label?"=TRUE, "Color"=T6 {"Red"=1.0, "Green"=0.0, "Blue"=1.0, "Alpha"=1.0}, "Radius"=sgl 1.0, "Length"=sgl 100.0, "Name"="Name") -> ("New Object Refnum"=w41:refnum<vi>)  [unwired: 3 in, 1 out]
      n13 = property class="SceneLight"(reference=w37, "Direction"=T4 {"X"=0.0, "Y"=0.0, "Z"=1.0} ("方向"), "Diffuse Color"=T5 {"Red"=0.1, "Green"=0.1, "Blue"=0.1, "Alpha"=0.1} ("散射光颜色"), "atInfinity"=TRUE ("位于无穷远处"), "Light Number"=0 ("光源编号"), "Position"=T4 {"X"=0.0, "Y"=0.0, "Z"=-10000.0} ("位置"), "Specular Color"=T5 {"Red"=0.0, "Green"=0.0, "Blue"=0.0, "Alpha"=0.0} ("反光颜色")) -> (reference out=w39:refnum<vi>)  [unwired: 1 in, 1 out]
      n14 = invoke class="SceneObject" method="Light.Add Light"(reference=w41, "Light"=w39) -> (reference out=w40:refnum<vi>)  [unwired: 2 in, 3 out]
      n15 = while {
        tunnel: w49 -> [w110]
        tunnel: w40 -> [w94]
        stop <- "?" stop-if-true
        # "Depth"
        # "ImageType_RGB8_Planar"
        n16 = call <userlib>:"MV3D RGBD Fetch Frame.vi"("nTimeOut"=u32 5000, "handle"=w110) -> ("function return"=→"fetchframe function":i32, "pstFrameData out"=w108:T11)  [unwired: 7 in, 1 out]
        n17 = Unbundle By Name(w108) -> ("MV3D_RGBD_IMAGE_DATA[0]"=w100:T12)
        n18 = Unbundle By Name(w108) -> ("MV3D_RGBD_IMAGE_DATA[1]"=w81:T12)
        n19 = Unbundle By Name(w100) -> ("nDataLen"=w106:u32)
        n20 = Unbundle By Name(w81) -> ("nDataLen"=w74:u32)
        n21 = Unbundle By Name(w100) -> ("nHeight"=w104:u32)
        n22 = Unbundle By Name(w100) -> ("nWidth"=w105:u32)
        n23 = Unbundle By Name(w81) -> ("nHeight"=w73:u32)
        n24 = Unbundle By Name(w100) -> ("pData"=w107:u32)
        n25 = Unbundle By Name(w81) -> ("pData"=w93:u32)
        n26 = Unbundle By Name(w81) -> ("nWidth"=w76:u32)
        n27 = call <userlib>:"MV3D RGBD Map Depth To Point Cloud.vi"("pstDepthImage"=w100, "handle"=w110) -> ("pstPointCloudImage out"=w54:T12, "function return"=→"depthtocloud return":i32)  [unwired: 6 in, 2 out]
        n28 = Unbundle By Name(w54) -> ("nDataLen"=w70:u32)
        n29 = Unbundle By Name(w54) -> ("pData"=w53:u32)
        n30 = dll-call lib="LabVIEW" fn="MoveBlock"("address"=w107, "size"=w106) -> ("value"=w103:i16[])  [unwired: 7 in, 2 out]
        n31 = Multiply(x=w73, y=w76) -> (x*y=w72:u32)
        n32 = dll-call lib="LabVIEW" fn="MoveBlock"("address"=w93, "value"=i16[] [] ("value 5"), "size"=w74) -> ("value"=w90:u8[])  [unwired: 6 in, 2 out]
        n33 = xnode "GetValueByPointer.xnode"("Pointer"=w53, "InputType"="InputType", "PackType"=T7."pack1") -> ("Output"=→"Output":cluster{string})  [unwired: 1 in, 1 out]
        n34 = Reshape Array(w103, w104, w105) -> (w102:i16[][])
        n35 = Divide(x=w70, y=u32 4) -> (x/y=w69:dbl)
        n36 = Multiply(x=w72, y=u32 2) -> (x*y=w92:u32)
        n37 = dll-call lib="LabVIEW" fn="MoveBlock"("address"=w53, "size"=w69) -> ("value"=w68:sgl[])  [unwired: 7 in, 2 out]
        n38 = Transpose 2D Array(2D array=w102) -> (transposed array=→"Depth":i16[][])
        n39 = Array Subset(array=w90, index=w72, length=w72) -> (w79:u8[])
        n40 = Array Subset(array=w90, index=w92, length=w72) -> (w78:u8[])
        n41 = To Unsigned Byte Integer(number=w79) -> (unsigned 8bit integer=w85:u8[])
        n42 = To Unsigned Byte Integer(number=w78) -> (unsigned 8bit integer=w82:u8[])
        n43 = Array Subset(array=w90, index=0 ("索引"), length=w72) -> (w80:u8[])
        n44 = Decimate 1D Array(w68) -> (w62:sgl[], w61:sgl[], w63:sgl[])
        n45 = Join Numbers(hi=w85, lo=w82) -> ((hi.lo)=w84:u16[])
        n46 = To Unsigned Byte Integer(number=w80) -> (unsigned 8bit integer=w83:u8[])
        n47 = Join Numbers(hi=w83, lo=w84) -> ((hi.lo)=w87:u32[])
        n48 = for {
          N: w72 -> [_]
          shift-right: [w145] -> w59
          shift-left: T5[] [] ("颜色数组") -> [w141]
          tunnel: w80 -> [w156] mode=indexing
          tunnel: w79 -> [w157] mode=indexing
          tunnel: w78 -> [w158] mode=indexing
          tunnel: w62 -> [w138] mode=indexing
          tunnel: w61 -> [w137] mode=indexing
          tunnel: w63 -> [w148] mode=indexing
          shift-right: [w146] -> w60
          shift-left: cluster{sgl, sgl, sgl}[] [] -> [w147]
          shift-right: [w139] -> w55
          shift-left: 0 ("x") -> [w140]
          w134 = sgl 1.0 ("y")
          # "PointCloud"
          n49 = Absolute Value(x=w138) -> (abs(x)=w136:sgl)
          n50 = Absolute Value(x=w137) -> (abs(x)=w135:sgl)
          n51 = Absolute Value(x=w148) -> (abs(x)=w149:sgl)
          n52 = To Single Precision Float(number=w156) -> (single precision float=w152:sgl)
          n53 = To Single Precision Float(number=w157) -> (single precision float=w154:sgl)
          n54 = To Single Precision Float(number=w158) -> (single precision float=w155:sgl)
          n55 = Less?(x=w136, y=w134) -> (x < y?=w133:bool)
          n56 = Less?(x=w135, y=w134) -> (x < y?=w132:bool)
          n57 = Less?(x=w149, y=w134) -> (x < y?=w131:bool)
          n58 = And(x=w133, y=w132) -> (x .and. y?=w130:bool)
          n59 = Divide(x=w152, y=255.0) -> (x/y=w144:dbl)
          n60 = And(x=w130, y=w131) -> (x .and. y?=w129:bool)
          n61 = Divide(x=w154, y=255.0) -> (x/y=w143:dbl)
          n62 = Divide(x=w155, y=sgl 255.0) -> (x/y=w142:sgl)
          n63 = case shown="真" w129 {
            tunnel: w138 -> [w174 _]
            tunnel: w137 -> [w173 _]
            tunnel: w148 -> [w172 _]
            tunnel: w147 -> [w170 w178]
            tunnel: [w169 w178] -> w146
            tunnel: [w168 w177] -> w145
            tunnel: w144 -> [w165 _]
            tunnel: w143 -> [w164 _]
            tunnel: w142 -> [w163 _]
            tunnel: w141 -> [w161 w177]
            tunnel: w140 -> [w160 w176]
            tunnel: [w159 w176] -> w139
            frame False {
              n64 = Bundle(cluster=cluster{sgl, sgl, sgl} {0.0, 0.0, 0.0} ("数组"), w174, w173, w172) -> (w171:cluster{sgl, sgl, sgl})
              n65 = Bundle By Name(cluster=T5 {"Red"=1.0, "Green"=1.0, "Blue"=0.0, "Alpha"=0.5} ("Color"), "Red"=w165, "Green"=w164, "Blue"=w163, "Alpha"=sgl 1.0) -> (w162:T5)
              n66 = Build Array (concatenate)(w170, w171) -> (w169:cluster{sgl, sgl, sgl}[])
              n67 = Increment(x=w160) -> (x+1=w159:i32)
              n68 = Build Array (concatenate)(w161, w162) -> (w168:T5[])
            }
            frame True {
            }
          }
        }
        "x+1" <- w55
        n69 = Reshape Array(w87, w73, w76) -> (w86:u32[][])
        n70 = call <vilib>:"Flatten Pixmap.vi"("24-bit pixmap"=w86) -> ("image data"=w71:T13)  [unwired: 10 in]
        n71 = call <vilib>:"Draw Flattened Pixmap.vi"("image data"=w71) -> ("new picture"=→"二维图片":picture)  [unwired: 8 in]
        n72 = for {
          N: w55 -> [_]
          tunnel: [w128] -> w58 mode=indexing
          i -> [w128]
        }
        n73 = Array Size(array=w59) -> (size(s)=→"大小":i32)
        n74 = call <vilib>:"Create Mesh.vi"() -> ("New Mesh Refnum"=w67:refnum<vi>)  [unwired: 10 in, 1 out]
        n75 = invoke class="SceneMesh" method="SetMeshParms"(reference=w67, "DrawMode"=T9."Points" ("绘图模式"), "VertArray"=w60, "Indices"=w58, "ColorMode"=T8."Per Vertex" ("颜色绑定模式"), "ColorArray"=w59) -> (reference out=w97:refnum<vi>)  [unwired: 5 in, 10 out]
        n76 = invoke class="SceneObject" method="Set Drawable"(reference=w94, "Drawable"=w97) -> (reference out=w66:refnum<vi>)  [unwired: 2 in, 3 out]
        n77 = invoke class="SceneObject" method="Transformation.Set Scale"(reference=w66, "Scale"=T4 {"X"=0.01, "Y"=0.01, "Z"=0.01} ("缩放")) -> (reference out=→"?":refnum<vi>)  [unwired: 2 in, 3 out]
      }
    }
    frame #4 {
      n78 = call <userlib>:"MV3D RGBD Stop.vi"("handle"=w180) -> ("function return"=→"stop function":i32, "handle out"=→"stop handle out":u32)  [unwired: 9 in]
    }
    frame #5 {
      n79 = call <userlib>:"MV3D RGBD Close Device.vi"("handle"=w183) -> ("function return"=→"close function":i32, "handle out"=→"close handle out":u32)  [unwired: 9 in]
    }
    frame #6 {
      n80 = call <userlib>:"MV3D RGBD Release.vi"() -> ("function return"=→"release function":i32)  [unwired: 11 in]
    }
  }
